vi "DR1 Camera Get Properties.vi"(9 "Session In":T1) -> (0 "Window_W":dbl=544.0, 1 "Height":dbl=200.0, 2 "DoubleRate_Enable":bool, 3 "Session Out":T1, 4 "WidthInterface":i64)   [LabVIEW 2012]
uses:
  <vilib>/userDefined/High Color/IMAQdx.ctl
  <resource>/objmgr/imaqdx.rc
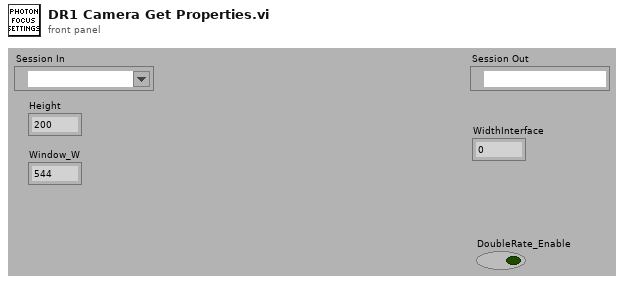
[diagram p1: front panel]
types:
  T1 = typedef "IMAQdx.ctl" = refnum<k21>
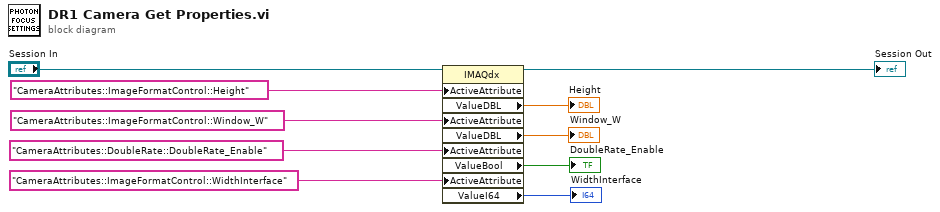
[diagram p0: block diagram]
diagram:
  n1 = property class="IMAQdx"(reference="Session In", "ActiveAttribute"="CameraAttributes::ImageFormatControl::Height", "ActiveAttribute"="CameraAttributes::ImageFormatControl::Window_W", "ActiveAttribute"="CameraAttributes::DoubleRate::DoubleRate_Enable", "ActiveAttribute"="CameraAttributes::ImageFormatControl::WidthInterface") -> (reference out=→"Session Out":T1, "ValueDBL"=→"Height":dbl, "ValueDBL"=→"Window_W":dbl, "ValueBool"=→"DoubleRate_Enable":bool, "ValueI64"=→"WidthInterface":i64)  [unwired: 1 in, 1 out]
